vi "Main.vi"() -> ()   [LabVIEW 2016]
doc: "The roboRIO Project template acquires acceleration data from the onboard accelerometer and displays the changes of acceleration values in a waveform chart."
uses:
  <vilib>/myRIO/Instrument Drivers/Onboard IO/DIO/typedefs/DIO Reference.ctl
  <vilib>/myRIO/Common/Instrument Driver Framework/Utilities/typedefs/myRIO Generic Hardware Reference.ctl
  <vilib>/myRIO/Common/Instrument Driver Framework/Utilities/typedefs/Hardware Version Enum.ctl
  <vilib>/myRIO/Common/Instrument Driver Framework/Utilities/typedefs/myRIO v1.0 Reference.ctl
  <vilib>/myRIO/Common/Instrument Driver Framework/Utilities/typedefs/Generic FPGA Reference.ctl
  <vilib>/myRIO/Common/Instrument Driver Framework/myRIO v1.0/DIO/typedefs/DIO Channels List.ctl
  <vilib>/myRIO/Common/Instrument Driver Framework/myRIO v1.0/DIO/typedefs/DIO Channels Enum.ctl
  <vilib>/userdefined/High Color/nirio_resource_hc.ctl
  <vilib>/Platform/TimedLoop/XDataNode/timing_clust.ctl
  <vilib>/Platform/TimedLoop/XDataNode/nitl_modes.ctl
  <vilib>/Platform/TimedLoop/XDataNode/wakeup.ctl
  <vilib>/myRIO/Common/Instrument Driver Framework/Utilities/vis/Is FPGA Ref Available.vi
  <vilib>/myRIO/Common/Instrument Driver Framework/roboRIO v1.0/DIO/vis/roboRIO v1.0 Open DIO.vi
  <vilib>/myRIO/Instrument Drivers/Onboard IO/DIO/vis/Write.vi
  <vilib>/myRIO/Common/Instrument Driver Framework/Utilities/vis/Validate Channels.vi
  <vilib>/myRIO/Common/Instrument Driver Framework/roboRIO v1.0/DIO/vis/roboRIO v1.0 Reserve DIO.vi
  <vilib>/myRIO/Common/Instrument Driver Framework/roboRIO v1.0/DIO/vis/roboRIO v1.0 Build MUX Configuration DIO.vi
  <vilib>/myRIO/Common/Instrument Driver Framework/roboRIO v1.0/Resource Manager/vis/roboRIO v1.0 Reserve Channel List.vi
  <vilib>/myRIO/Common/Instrument Driver Framework/roboRIO v1.0/Resource Manager/vis/roboRIO v1.0 Create Configuration List.vi
  <vilib>/myRIO/Common/Instrument Driver Framework/roboRIO v1.0/Resource Manager/vis/roboRIO v1.0 Reserve Channel.vi
  <vilib>/myRIO/Common/Instrument Driver Framework/roboRIO v1.0/Resource Manager/vis/roboRIO v1.0 Unreserve Channel.vi
  <vilib>/myRIO/Common/Instrument Driver Framework/roboRIO v1.0/Resource Manager/vis/roboRIO v1.0 Build Mutex Name.vi
  <vilib>/FPGAPlugInAG/roboRIO/niLvFpga_Open_roboRIO.vi
  <vilib>/rvi/interface/common/dynamic/niFpgaDynamicAddResources.vi
  <vilib>/FPGAPlugInAG/Dynamic/niLvFpga_Reset_Dynamic.vi
  <vilib>/Utility/VariantDataType/GetNumericInfo.vi
  <vilib>/Utility/error.llb/Error Cluster From Error Code.vi
  <vilib>/myRIO/Common/Instrument Driver Framework/roboRIO v1.0/roboRIO v1.0 Open.vi
  <vilib>/myRIO/Common/Instrument Driver Framework/Utilities/vis/IO Manager.vi
  <vilib>/myRIO/Common/Instrument Driver Framework/Utilities/vis/Configuration Manager.vi
  <vilib>/myRIO/Common/Instrument Driver Framework/roboRIO v1.0/Resource Manager/vis/roboRIO v1.0 Configure IO.vi
  <vilib>/myRIO/Common/Instrument Driver Framework/myRIO v1.0/myRIO v1.0 Close.vi
  <vilib>/myRIO/Common/Instrument Driver Framework/roboRIO v1.0/DIO/vis/roboRIO v1.0 Write DIO.vi
  <vilib>/FPGAPlugInAG/Dynamic/niLvFpga_Run_Dynamic.vi
  <vilib>/rvi/errors/niLvFpgaAdjustHostInterfaceError.vi
  <vilib>/rvi/interface/nirviOpenFPGA/nirviOpenFPGA.xnode
  FPGA Bitfiles/AutoBikeProject_FPGATarget_AutoBikeFPGA_EwzLm8KNttI.lvbitx
  <vilib>/rvi/interface/nirviMethod/nirviMethod.xnode
  <vilib>/myRIO/Express VI/Onboard Devices/LED/LED Express VI.xnode
  <vilib>/myRIO/Instrument Drivers/Onboard IO/DIO/vis/myRIO DIO Open.xnode
  <vilib>/rvi/interface/nirviReadWriteControl/nirviReadWriteControl.xnode
  <vilib>/Platform/TimedLoop/XDataNode/XDataNode.xnode
  <vilib>/Platform/TimedLoop/XDataNode/XDNodeRunTimeDep.lvlib
  <vilib>/rvi/interface/Simulation/niFpgaSimulationCallBeginRW.vi
  <vilib>/addons/Fuzzy Logic/NI_Fuzzy_Logic_API.lvlib
  <vilib>/myRIO/Instrument Drivers/Onboard IO/DIO/DIO.lvlib
  NiFpgaLv.dll
panel:
  in  "Number of bias loops":i32=1000
  in  "Calc bias":bool
  in  "Stop Button":bool
  in  "Reference Speed":sgl=8.0
  in  "Front Panel Steering Duty Cycle":dbl(slide) scale=0.0..1.0
  in  "error in (no error)":errorcluster
  in  "Steering direction":bool
  in  "Color Box 2":u32(colorbox)
  out "Roll(deg)":dbl
  out "Steering angle (deg)":dbl
  out "Duty cycle":dbl
  out "Iteration duration":i64
  out "Current velocity":dbl
  out "Main loop lates":i32
  out "Error out main loop":errorcluster
  out "Main loop finish late":bool
  in  "Color Box":u32(colorbox)
  # "INPUTS"
  # "CW"
  # "CC"
  # "OUTPUTS"
  # "Main loop timing"
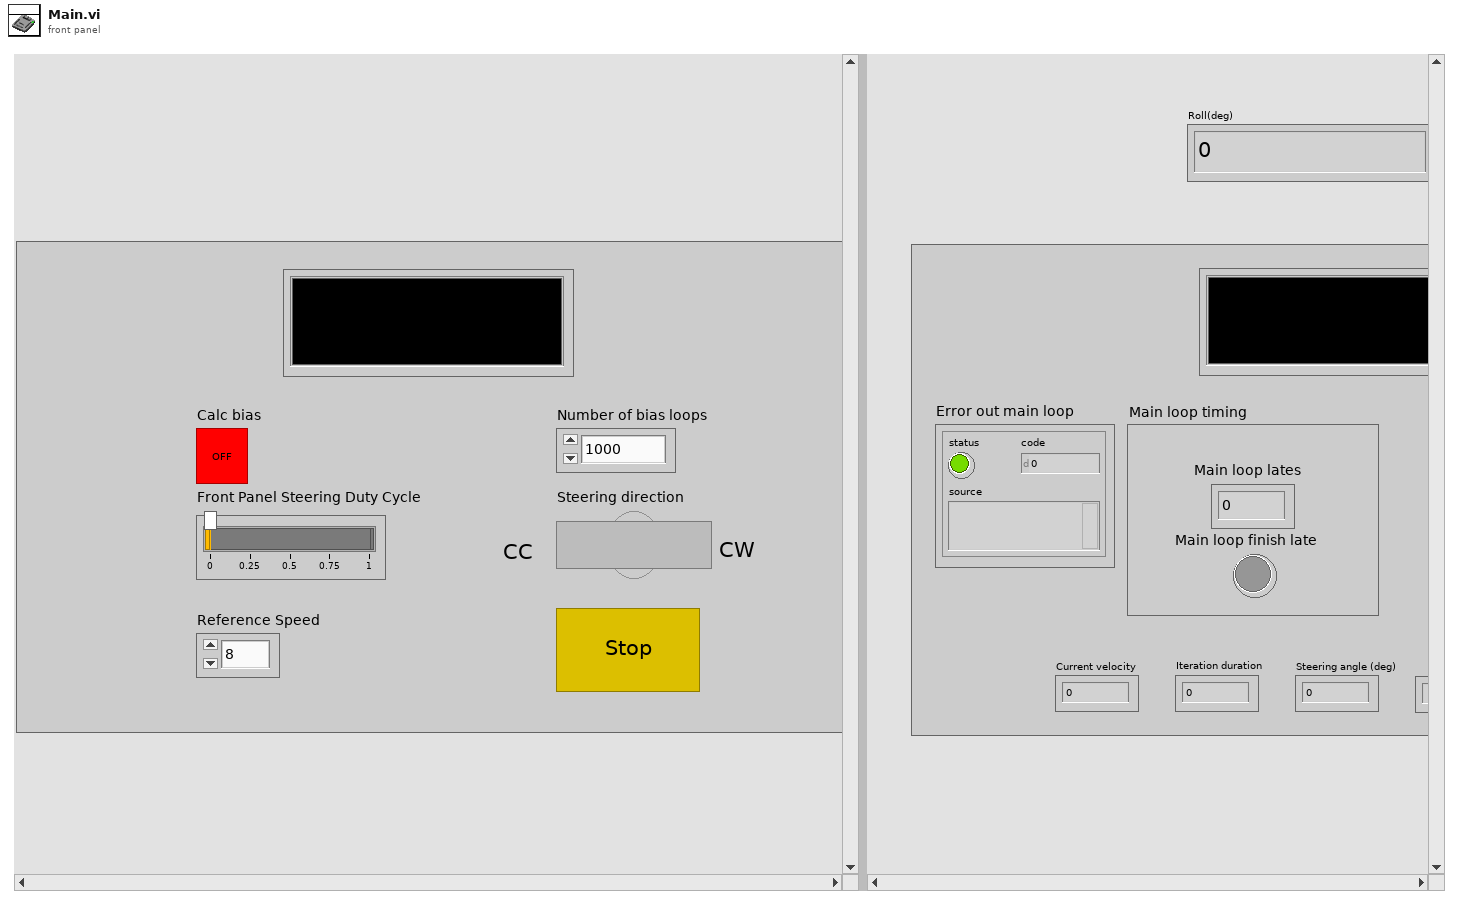
[diagram p1: front panel]
types:
  T1 = typedef "DIO.lvlib/DIO Reference.ctl" = cluster{"myRIO Reference":T2, "DIO Channels List":T6}
  T2 = typedef "myRIO Generic Hardware Reference.ctl" = cluster{"myRIO Model":T3, "myRIO Hardware Reference":T4}
  T3 = typedef "Hardware Version Enum.ctl" = enum16{"Unknown", "myRIO-1900", "myRIO-1950", "roboRIO", "NI ELVIS RIO CM"}
  T4 = typedef "myRIO v1.0 Reference.ctl" = cluster{"Generic FPGA Reference":T5, "Allow multiple opens":bool}
  T5 = typedef "Generic FPGA Reference.ctl" = refnum<k20>
  T6 = typedef "DIO Channels List.ctl" = T7[]
  T7 = typedef "DIO Channels Enum.ctl" = enum16{"Not Connected", "C/DIO0", "C/DIO1", "C/DIO2", "C/DIO3", "C/DIO4", "C/DIO5", "C/DIO6", "C/DIO7", "A/DIO0", "A/DIO1", "A/DIO2", "A/DIO3", "A/DIO4", "A/DIO5", "A/DIO6", "A/DIO7", "A/DIO8", "A/DIO9", "A/DIO10", "A/DIO11", "A/DIO12", "A/DIO13", "A/DIO14", "A/DIO15", "B/DIO0", "B/DIO1", "B/DIO2", "B/DIO3", "B/DIO4", "B/DIO5", "B/DIO6", "B/DIO7", "B/DIO8", "B/DIO9", "B/DIO10", "B/DIO11", "B/DIO12", "B/DIO13", "B/DIO14", "B/DIO15", "LED0", "LED1", "LED2", "LED3", "Button0", "DIO/DIO0", "DIO/DIO1", "DIO/DIO2", "DIO/DIO3", "DIO/DIO4", "DIO/DIO5", "DIO/DIO6", "DIO/DIO7", "DIO/DIO8", "DIO/DIO9", "SPI/CS0", "SPI/CS1", "SPI/CS2", "SPI/CS3", "LED RADIO (Green)", "LED RADIO (Red)", "LED COMM (Green)", "LED COMM (Red)", "LED MODE (Green)", "LED MODE (Red)"}
  T8 = typedef "nirio_resource_hc.ctl" = tag
  T9 = enum16{"open", "open or create", "create or replace", "create", "open (read-only)"}
  T10 = cluster{"FilteredGyroX":dbl, "FilteredGyroY":dbl}
  T11 = typedef "XDNodeRunTimeDep.lvlib/timing_clust.ctl" = cluster{"Expected End [f-1]":u64, "Actual End [f-1]":u64, "Finished Late? [f-1]":bool, "Expected End [i-1]":u64, "Actual End [i-1]":u64, "Finished Late? [i-1]":bool, "Expected Start [i]":u64, "Actual Start [i]":u64, "Expected Start [f]":u64, "Actual Start [f]":u64, "Source Name":string, "Structure Name":string, "Period":i64, "Deadline":i64, "Offset":i64, "Start":i64, "Priority":i32, "Timeout":i32, "Mode":T12, "Wakeup Reason":T13, "Error":errorcluster, "Source Type":string, "Secondary Source Type":string, "Global End Time":u64, "Global Start Time":u64, "Frame Duration":u64, "Iteration Duration":u64, "Assigned CPU":i32, "I/O Scan Engine Mode":u32}
  T12 = typedef "XDNodeRunTimeDep.lvlib/nitl_modes.ctl" = enum32{"No Change", "Process missed periods, maintain original phase", "Discard missed periods, maintain original phase", "Process missed periods, ignore original phase", "Discard missed periods, ignore original phase"}
  T13 = typedef "XDNodeRunTimeDep.lvlib/wakeup.ctl" = enum32{"Normal", "Aborted", "Asynchronous wakeup", "Timing source error", "Timed loop error", "Timeout"}
  T14 = cluster{"X gyro bias":dbl, "Y gyro bias":dbl, "Z gyro bias":dbl, "X acc bias":dbl, "Y acc bias":dbl, "Z acc bias":dbl}
  T15 = cluster{"B":dbl[][], "Cline":dbl[][], "Kline":dbl[][], "Mline":dbl[][], "Alp0":dbl, "Alp1":dbl, "Gam0":dbl, "Gam1":dbl, "T_shift":dbl, "Numerator":dbl[], "Denominator":dbl[]}
  T16 = typedef "NI_LinSys_Model Typedefs.lvlib/CD State Space Model (MIMO).ctl" = cluster{"properties":T17, "A":dbl[][], "B":dbl[][], "C":dbl[][], "D":dbl[][], "StateNames":string[], "Transport Delay":dbl[][]}
  T17 = typedef "NI_LinSys_Model Typedefs.lvlib/CD General Elements.ctl" = cluster{"Model name":string, "Input names":string[], "Output names":string[], "Input Delays":dbl[], "Output Delays":dbl[], "Sampling Time":dbl, "Notes":string}
  T18 = typedef "NI_LinSys_Model Typedefs.lvlib/CD Transfer Function Model (MIMO).ctl" = cluster{"properties":T17, "transfer function(s)":T19[][]}
  T19 = typedef "NI_LinSys_Model Typedefs.lvlib/CD Transfer Function Model (SISO).ctl" = cluster{"Numerator":dbl[], "Denominator":dbl[], "delay":dbl}
  T20 = cluster{"SysD":T16, "sysDo":T16, "sysDi":T16, "sysDC":T18}
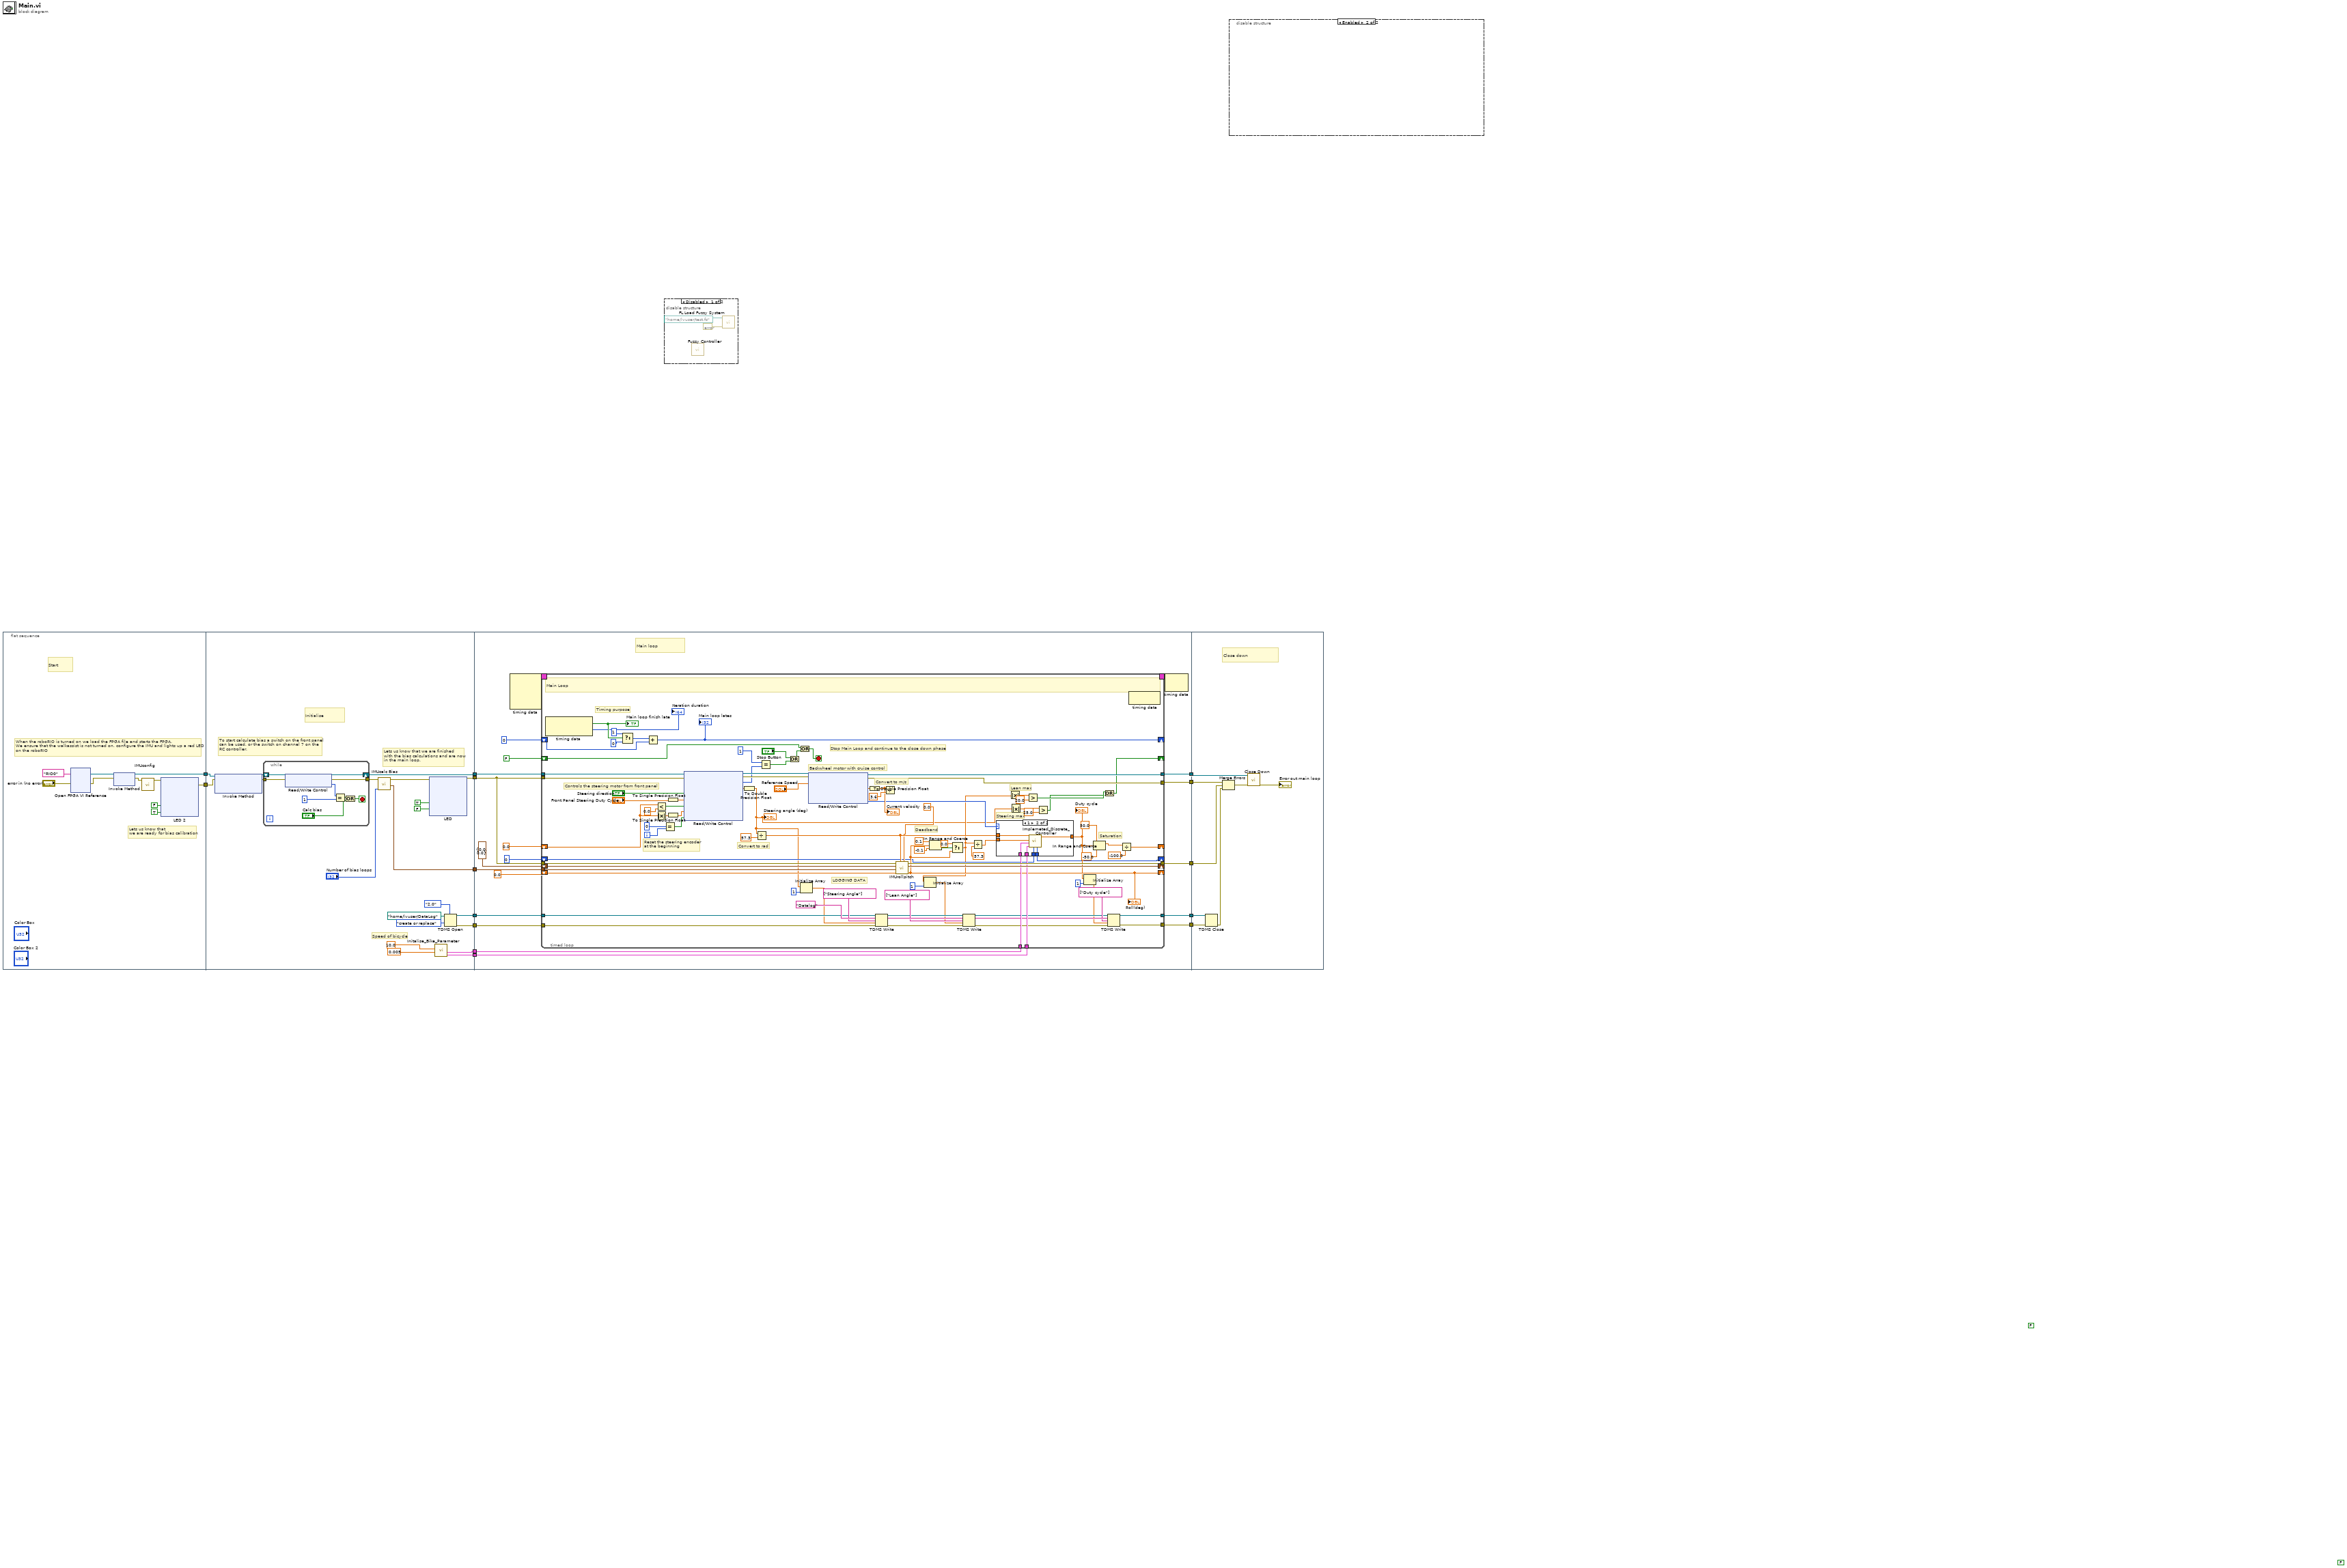
[diagram p0: block diagram]
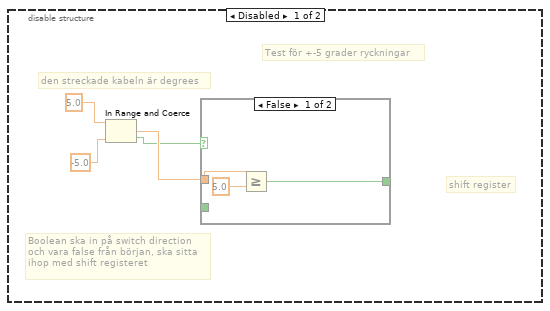
[diagram p3: hidden frame]
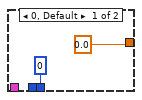
[diagram p5: hidden frame]
diagram:
  (unwired) FALSE
  (unwired) FALSE
  n1 = flat-sequence {
    tunnel: [w17] -> w11
    tunnel: [w16] -> w10
    tunnel: [w74] -> w14
    tunnel: [w78] -> w13
    tunnel: w11 -> [w77]
    tunnel: w10 -> [w71]
    tunnel: [w70] -> w9
    tunnel: [w67] -> w8
    tunnel: [w66] -> w7
    tunnel: [w62] -> w6
    tunnel: [w61] -> w5
    tunnel: w14 -> [w146]
    tunnel: w13 -> [w140]
    tunnel: [w145] -> w12
    tunnel: w9 -> [w141]
    tunnel: w8 -> [w136]
    tunnel: w7 -> [w135]
    tunnel: w6 -> [w134]
    tunnel: w5 -> [w133]
    tunnel: [w132] -> w4
    tunnel: [w131] -> w3
    tunnel: [w130] -> w2
    tunnel: [w129] -> w1
    tunnel: w12 -> [w260]
    tunnel: w4 -> [w257]
    tunnel: w3 -> [w256]
    tunnel: w2 -> [w255]
    tunnel: w1 -> [w254]
    frame #0 {
      # "Start"
      # "Lets us know that\nwe are ready for bias calibration"
      # "When the roboRIO is turned on we load the FPGA file and starts the FPGA.\nWe ensure that the walkassist is not turned on, configure the IMU and lights up a red LED\non the roboRIO"
      n2 = xnode "Open FPGA VI Reference"("error in"="error in (no error)", "resource name"=tag "RIO0") -> ("FPGA VI Reference Out"=w23:refnum<k20>, "error out"=w24:errorcluster)
      n3 = xnode "Invoke Method"("FPGA VI Reference In"=w23, "error in"=w24) -> ("FPGA VI Reference Out"=w16:refnum<k20>, "error out"=w15:errorcluster)
      n4 = call "IMUconfig.vi"("error in (no error)"=w15) -> ("error out"=w18:errorcluster)  [unwired: 10 in]
      n5 = xnode "LED 2"("COMM (Green)"=FALSE, "COMM (Red)"=TRUE, "error in (no error)"=w18) -> ("error out"=w17:errorcluster)
    }
    frame #1 {
      # "Speed of bicycle"
      # "Lets us know that we are finished\nwith the bias calculations and are now\nin the main loop."
      # "To start calculate bias a switch on the front panel\ncan be used, or the switch on channel 7 on the \nRC controller."
      # "Initialise"
      n6 = xnode "Invoke Method"("FPGA VI Reference In"=w71, "error in"=w77) -> ("FPGA VI Reference Out"=w76:refnum<k20>, "error out"=w75:errorcluster)  [unwired: 1 in]
      n7 = while {
        tunnel: w75 -> [w89]
        shift-right: [w88] -> w74
        shift-left: w76 -> [w90]
        tunnel: [w87] -> w73
        stop <- w83 stop-if-true
        n8 = xnode "Read/Write Control"("FPGA VI Reference In"=w90, "error in"=w89) -> ("FPGA VI Reference Out"=w88:refnum<k20>, "error out"=w87:errorcluster, "Channel 7 position"=w86:i32)
        n9 = Equal?(x=w86, y=1) -> (x = y?=w84:bool)
        n10 = Or(x=w84, y="Calc bias") -> (x .or. y?=w83:bool)
      }
      n11 = call "IMUcalc Bias.vi"("Number of loops"="Number of bias loops", "error in (no error)"=w73) -> ("Bias"=w70:T14, "error out"=w72:errorcluster)  [unwired: 7 in]
      n12 = xnode "LED"("COMM (Green)"=TRUE, "COMM (Red)"=FALSE, "error in (no error)"=w72) -> ("error out"=w78:errorcluster)
      n13 = call "Initalise_Bike_Parameter.vi"("Ts"=0.005, "Velocity"=10.0) -> ("Other variables"=w67:T15, "systems"=w66:T20)  [unwired: 7 in]
      n14 = TDMS Open(7:enum16{"1.0", "2.0"}."2.0" ("file format version (2.0)"), 10:T9."create or replace" ("operation (0:open)"), 11:path "/home/lvuser/DataLog" ("file path")) -> (0:w62:errorcluster, 3:w61:refnum<k34>)  [unwired: 4 in]
    }
    frame #2 {
      # "Main loop"
      n15 = node-c288() -> (w144:T11)  [unwired: 4 in]
      n16 = timed-loop {
        timing: w144 -> [_]
        timing-out: [_] -> w143
        tunnel: w140 -> [w230]
        tunnel: [w236] -> w145
        tunnel: w146 -> [w231]
        tunnel: [w211] -> w131
        shift-right: [w195] -> _
        shift-left: 0.0 -> [w232]
        shift-right: [w213] -> _
        shift-left: 0 -> [w212]
        tunnel: w141 -> [w209]
        tunnel: w140 -> [w188]
        shift-right: [w205] -> _
        shift-left: T10 {"FilteredGyroX"=0.0, "FilteredGyroY"=0.0} ("FilteredGyro(deg)") -> [w206]
        shift-right: [w170] -> _
        shift-left: 0.0 ("Roll(deg)") -> [w204]
        tunnel: [w202] -> w132
        tunnel: w136 -> [w200]
        tunnel: w135 -> [w199]
        tunnel: w134 -> [w185]
        tunnel: w133 -> [w184]
        tunnel: [w181] -> w130
        tunnel: [w180] -> w129
        shift-right: [w160] -> _
        shift-left: 0 ("Loop Out") -> [w159]
        shift-right: [w150] -> _
        shift-left: FALSE -> [w147]
        i -> [w237]
        stop <- w148 stop-if-true
        # "Steering max"
        # "Lean max"
        # "Saturation"
        # "Stop Main Loop and continue to the close down phase"
        # "Deadband"
        # "LOGGING DATA"
        # "Convert to m/s"
        # "Convert to rad"
        # "Reset the steering encoder\nat the beginning"
        # "Controls the steering motor from front panel"
        # "Backwheel motor with cruise control"
        # "Timing purpose"
        # "Main Loop"
        n17 = node-c288() -> (w217:bool, →"Iteration duration":i64)  [unwired: 1 in]
        "Main loop finish late" <- w217
        n18 = Select(t=1, s=w217, f=0) -> (s? t:f=w215:i32)
        n19 = Add(x=w215, y=w212) -> (x+y=w213:i32)
        "Main loop lates" <- w213
        n20 = Less?(x=w232, y=0.0) -> (x < y?=w222:bool)
        n21 = Absolute Value(x=w232) -> (abs(x)=w221:dbl)
        n22 = Equal?(x=0, y=w237) -> (x = y?=w219:bool)
        n23 = To Single Precision Float(number="Front Panel Steering Duty Cycle") -> (single precision float=w224:sgl)
        n24 = To Single Precision Float(number=w221) -> (single precision float=w220:sgl)
        n25 = xnode "Read/Write Control"("FPGA VI Reference In"=w231, "error in"=w230, "Front Panel Direction"="Steering direction", "Front Panel Duty Cycle"=w224, "Control Loop Direction"=w222, "Control Loop Duty Cycle"=w220, "Reset counter"=w219) -> ("FPGA VI Reference Out"=w228:refnum<k20>, "error out"=w227:errorcluster, "Channel 4 position"=w218:i32, "Steering angle(deg)"=w208:sgl)
        n26 = To Double Precision Float(number=w208) -> (double precision float=w155:dbl)
        "Steering angle (deg)" <- w155
        n27 = Divide(x=w155, y=57.3) -> (x/y=w163:dbl)
        n28 = Equal?(x=1 ("y"), y=w218) -> (x = y?=w235:bool)
        n29 = Or(x="Stop Button", y=w235) -> (x .or. y?=w149:bool)
        n30 = Or(x=w147, y=w149) -> (x .or. y?=w148:bool)
        n31 = Initialize Array(w155, 1 ("dimension size")) -> (w177:dbl[])
        n32 = xnode "Read/Write Control"("FPGA VI Reference In"=w228, "error in"=w227, "Reference speed in km/h"="Reference Speed") -> ("FPGA VI Reference Out"=w236:refnum<k20>, "error out"=w211:errorcluster, "Current speed"=w229:sgl, "Channel 6 position"=w161:i32)  [unwired: 1 out]
        n33 = To Double Precision Float(number=w229) -> (double precision float=w197:dbl)
        "Current velocity" <- w197
        n34 = TDMS Write(0:w184, 5:"Datalog" ("group name in (Untitled)"), 7:string[] ["Steering Angle"] ("channel name(s) in (Untitled)"), 9:w177, 11:w185) -> (4:w183:refnum<k34>, 6:w192:string, 15:w187:errorcluster)  [unwired: 1 in, 1 out]
        n35 = Divide(x=w197, y=3.6) -> ()  [unwired: 1 out]
        n36 = call "IMUrollpitch.vi"("v(m/s)"=0.0, "SteeringAngle(rad/s)"=w163, "PrevRoll(deg)"=w204, "Bias"=w209, "PrevFilteredGyro(deg)"=w206, "error in (no error)"=w188) -> ("Roll(deg)"=w170:dbl, "FilteredGyro(deg)"=w205:T10, "error out"=w202:errorcluster)  [unwired: 3 in]
        "Roll(deg)" <- w170
        n37 = In Range and Coerce(upper limit=0.1, x=w170, lower limit=-0.1) -> (In Range?=w171:bool)  [unwired: 1 out]
        n38 = Select(t=0.0, s=w171, f=w170) -> (s? t:f=w157:dbl)
        n39 = Initialize Array(w157, 1 ("dimension size")) -> (w176:dbl[])
        n40 = TDMS Write(0:w183, 5:w192, 7:string[] ["Lean Angle"] ("channel name(s) in (Untitled)"), 9:w176, 11:w187) -> (4:w182:refnum<k34>, 6:w191:string, 15:w186:errorcluster)  [unwired: 1 in, 1 out]
        n41 = Divide(x=w157, y=57.3) -> (x/y=w164:dbl)
        n42 = case shown="1" w161 {
          tunnel: w200 -> [_ w247]
          tunnel: w199 -> [_ w246]
          tunnel: [0.0 w245] -> w167
          tunnel: w164 -> [_ w244]
          tunnel: w163 -> [_ w243]
          tunnel: [0 ("Loop Out") w242] -> w160
          tunnel: w159 -> [_ w241]
          frame 0, Default {
          }
          frame 1 {
            n43 = call "Implemeted_Discrete_Controller.vi"("Loop Itr"=w241, "Other variables"=w247, "systems"=w246, "Lean Angle"=w244, "Steer Angle"=w243) -> ("Duty Cycle"=w245:dbl, "Loop Out"=w242:i32)  [unwired: 4 in, 1 out]
          }
        }
        "Duty cycle" <- w167
        n44 = Absolute Value(x=w157) -> (abs(x)=w158:dbl)
        n45 = Absolute Value(x=w155) -> (abs(x)=w156:dbl)
        n46 = Greater?(x=w158, y=20.0) -> (0:w152:bool)
        n47 = Greater?(x=w156, y=25.0) -> (0:w151:bool)
        n48 = Initialize Array(w167, 1 ("dimension size")) -> (w174:dbl[])
        n49 = In Range and Coerce(upper limit=50.0, x=w167, lower limit=-50.0) -> (coerced(x)=w168:dbl)  [unwired: 1 out]
        n50 = Or(x=w152, y=w151) -> (x .or. y?=w150:bool)
        n51 = TDMS Write(0:w182, 5:w191, 7:string[] ["Duty cycle"] ("channel name(s) in (Untitled)"), 9:w174, 11:w186) -> (4:w181:refnum<k34>, 15:w180:errorcluster)  [unwired: 1 in, 2 out]
        n52 = Divide(x=w168, y=-100.0) -> (x/y=w195:dbl)
        n53 = node-c288() -> ()  [unwired: 1 in, 1 out]
      }
      n54 = node-c288(w143) -> ()  [unwired: 1 out]
    }
    frame #3 {
      # "Close down"
      n55 = TDMS Close(8:w254, 11:w255) -> (0:w258:errorcluster)  [unwired: 1 out]
      n56 = Merge Errors(w256, w257, w258) -> (w259:errorcluster)
      n57 = call "Close Down.vi"("error in (no error)"=w259, "FPGA VI Reference Out"=w260) -> ("error out"=→"Error out main loop":errorcluster)  [unwired: 9 in]
    }
  }
  n58 = disable-structure shown="Disabled" {
    frame Disabled {
      n59 = call "Fuzzy Controller.vi"() -> ()  [unwired: 10 in, 2 out]
      n60 = call <vilib>:"FL Load Fuzzy System.vi"("error in (no error)"=errorcluster {"status"=FALSE, "code"=0, "source"=""}, "file path"=path "/home/lvuser/test.fs") -> ()  [unwired: 8 in, 2 out]
    }
    frame Enabled {
    }
  }
  n61 = disable-structure shown="Enabled" {
    frame Disabled {
      # "Test för +-5 grader ryckningar"
      # "den streckade kabeln är degrees"
      # "Boolean ska in på switch direction\noch vara false från början, ska sitta\nihop med shift registeret"
      # "shift register"
      n62 = In Range and Coerce(upper limit=5.0, lower limit=-5.0) -> (x=w267:dbl, In Range?=w266:bool)  [unwired: 1 out]
      n63 = case shown="False" w266 {
        tunnel: w267 -> [w270 _]
        tunnel: [w268 w271] -> _
        tunnel: _ -> [_ w271]
        frame False {
          n64 = Greater Or Equal?(x=w270, y=5.0) -> (x >= y?=w268:bool)
        }
        frame True {
        }
      }
    }
    frame Enabled {
    }
  }
